vi "set wave form.vi"(10 "channels (0)":string[](array[string])=["0"], 11 "device (1)":i16=1) -> (0 "plot labels":T3, 1 "last value":dbl[](array[numeric]) format="%.2f", 2 "waveforms":T4 format="%.2f", 3 "SD method out":T2={"method array"=[], "Method Description"="", "data frequency"=1200, "repeat period"=2400} {"method array"."offset" format="%.2f"; "method array"."amplitude" format="%.2f"; "method array"."cycles/repeat period" min=1})   [LabVIEW 2010]
uses:
  wavecluster.ctl
  SDMethod.ctl
  plot labels.ctl
panel:
  in  "zoom control":T1(ring)=enum."Show repeat period"
  out "Time between Cursors":dbl format="%.4f"
  in  "show cycles":u32=1 min=1
  out "actual ticks per second":sgl format="%.8f"
  out "tick length":sgl=0.8333334 format="%.8f"
  in  "SD method default":T2 {"method array"."offset" format="%.2f"; "method array"."amplitude" format="%.2f"; "method array"."cycles/repeat period" min=1}
  out "channel label":string
  out "ticks/cycle":sgl=inf format="%.2f"
  out "integer":bool
  out "channel frequency":sgl format="%.8f"
  out "overall frequency":sgl=0.5 format="%.8f"
  in  "color":u32[](array[colorbox])=[255, 16711680, 52275, 16776960, 16750848, 16724991, 65535, 16777215]
  in  "load method":bool
  in  "save method":bool
  in  "SD method":T2={"method array"=[], "Method Description"="", "data frequency"=1200, "repeat period"=2400} {"method array"."waveform" items=["none", "one", "two", "3", "4", "5", "6", "7"]; "method array"."offset" format="%.2f"; "method array"."amplitude" format="%.2f"; "method array"."cycles/repeat period" min=1}
  in  "stop":bool
  out "graph":cluster{i32, sgl, "waveforms out":sgl[][]}(graph)={0, 0.00083333335, "waveforms out"=[]}
  # "ms"
  # "hz"
  # "ticks"
  # "hz"
  # "ms"
  # "hz"
  # "ticks"
  # "hz"
  # "ticks"
  # "ticks"
  # "volts"
  # "volts"
  # "ticks"
  # "hz"
  # "ticks"
  # "ticks"
  # "volts"
  # "volts"
  # "ticks"
  # "hz"
  # "ticks"
  # "ticks"
  # "volts"
  # "volts"
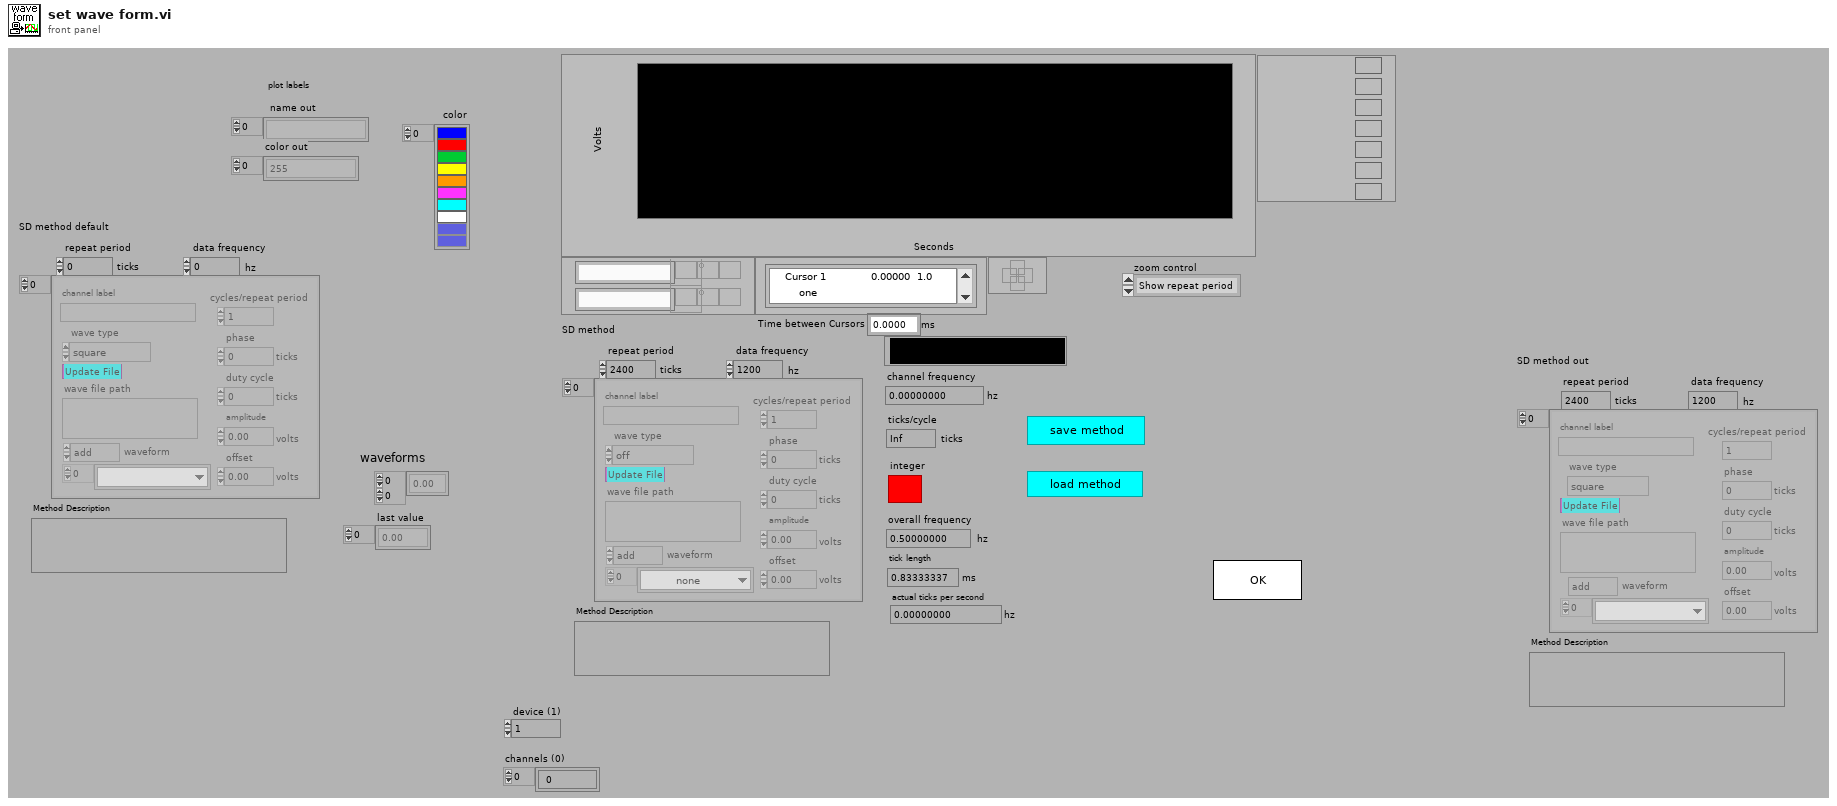
[diagram p1: front panel]
types:
  T1 = enum16{"Use zoom controls", "Show repeat period", "Show cycle"}
  T2 = typedef "SDMethod.ctl" = cluster{"method array":cluster{"wave type":enum16{"off", "square", "sine", "triangle", "sawtooth", "from file", "wavemaker", "flume pump"}, "cycles/repeat period":u32, "phase":i32, "duty cycle":u32, "wave file path":path, "amplitude":dbl, "channel label":string, "Update":bool, "offset":dbl, " waveform":u16[], "Function":enum16{"add", "multiply"}}[], "Method Description":string, "data frequency":u32, "repeat period":u32}
  T3 = typedef "plot labels.ctl" = cluster{"name out":string[], "color out":u32[]}
  T4 = typedef "wavecluster.ctl" = sgl[][]
  T5 = cluster{"wave type":enum16{"off", "square", "sine", "triangle", "sawtooth", "from file", "wavemaker", "flume pump"}, "cycles/repeat period":u32, "phase":i32, "duty cycle":u32, "wave file path":path, "amplitude":dbl, "channel label":string, "Update":bool, "offset":dbl, " waveform":u16[], "Function":enum16{"add", "multiply"}}[]
  T6 = cluster{"ticks per second used":sgl, "seconds per tick used":sgl, "timebase signal used":sgl, "timebase divisor used":i32}
  T7 = cluster{"wave type":enum16{"off", "square", "sine", "triangle", "sawtooth", "from file", "wavemaker", "flume pump"}, "cycles/repeat period":u32, "phase":i32, "duty cycle":u32, "wave file path":path, "amplitude":dbl, "channel label":string, "Update":bool, "offset":dbl, " waveform":u16[], "Function":enum16{"add", "multiply"}}
  T8 = enum16{"off", "square", "sine", "triangle", "sawtooth", "from file", "wavemaker", "flume pump"}
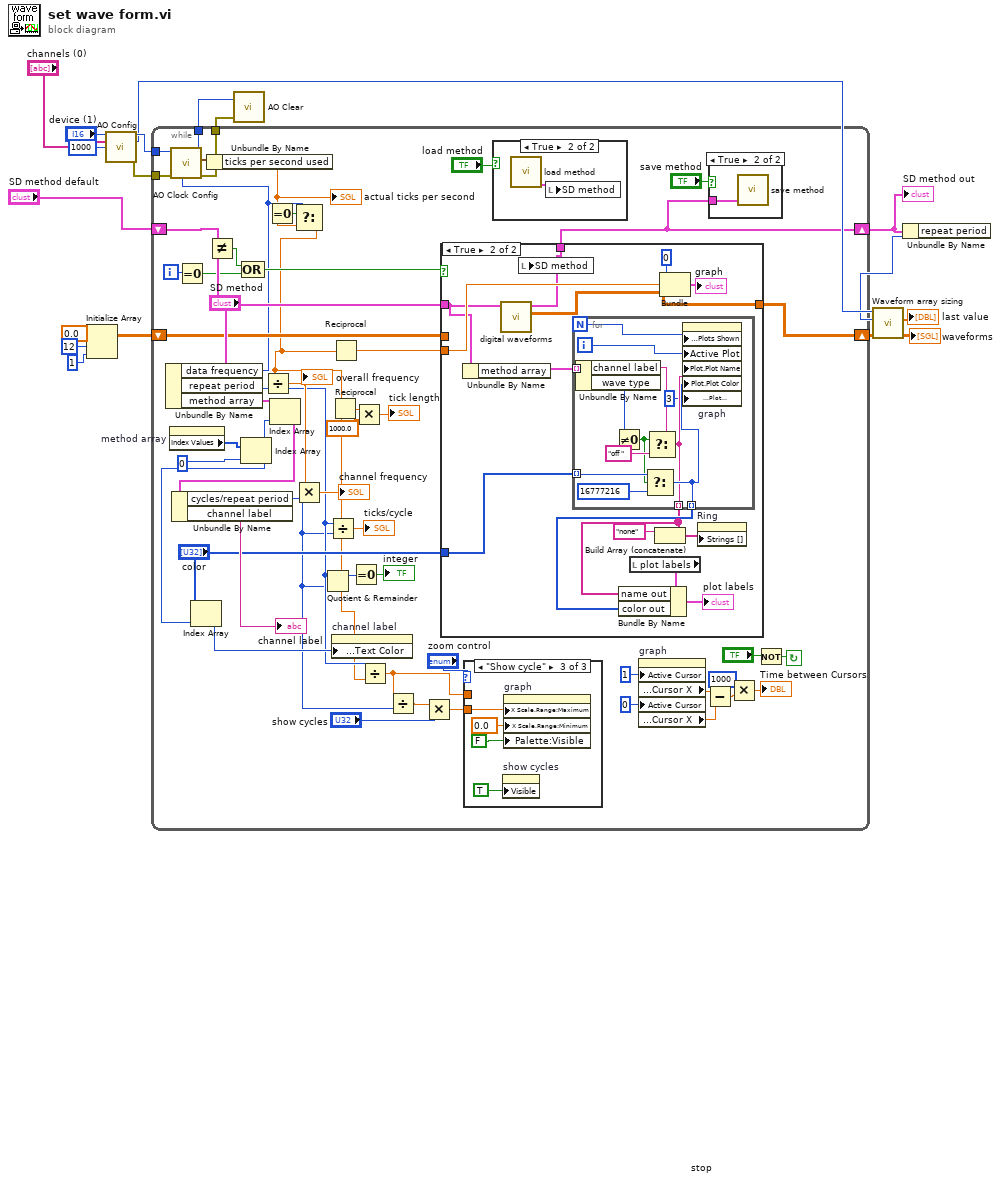
[diagram p0: block diagram]
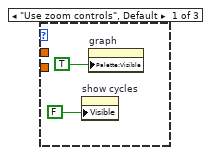
[diagram p2: hidden frame]
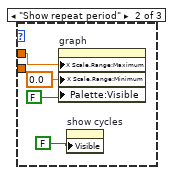
[diagram p3: hidden frame]
diagram:
  n1 = Initialize Array(sgl 0.0, 12, 1) -> (w16:sgl[][])
  n2 = call "AO Config.vi"("device (1)"="device (1)", "channels (0)"="channels (0)", "buffer size (1000 updates)"=1000) -> ("taskID"=w9:u32, "number of channels"=w3:u32, "error out"=w10:errorcluster)  [unwired: 10 in]
  n3 = while {
    tunnel: [w40] -> w7
    tunnel: [w41] -> w8
    tunnel: w9 -> [w44]
    tunnel: w10 -> [w42]
    shift-left: w16 -> [w58]
    shift-right: [w69] -> w4
    shift-left: "SD method default" -> [w64]
    shift-right: [w60] -> w14
    i -> [w68]
    stop <- w70 continue-if-true
    n4 = Unbundle By Name("SD method") -> ("data frequency"=w34:u32, "repeat period"=w39:u32, "method array"=w56:T5)
    n5 = property on="method array" class="Arr"() -> ("Index Values"=w29:u32[])  [unwired: 2 in, 2 out]
    n6 = call "AO Clock Config.vi"("ticks per second (-1: no change)"=w34, "error in (no error)"=w42, "task ID"=w44) -> ("error out"=w40:errorcluster, "actual rates used"=w43:T6, "task ID out"=w41:u32)  [unwired: 6 in]
    n7 = Equal To 0?(x=w68) -> (x = 0?=w59:bool)
    n8 = Unbundle By Name(w43) -> ("ticks per second used"=w33:sgl)
    "actual ticks per second" <- w33
    n9 = Not Equal?(x=w64, y="SD method") -> (x != y?=w67:bool)
    n10 = Index Array(array=w29, index=0) -> (element=w30:u32)
    n11 = Index Array(array="color", index=w30) -> (element=w49:u32)
    n12 = Compound Arithmetic op=OR(w67, w59) -> (w62:bool)
    n13 = Equal To 0?(x=w33) -> (x = 0?=w31:bool)
    n14 = Index Array(array=w56, index=w30) -> (element=w55:T7)
    n15 = Unbundle By Name(w55) -> ("cycles/repeat period"=w36:u32, "channel label"=→"channel label":string)
    n16 = Select(t=w34, s=w31, f=w33) -> (s? t:f=w32:sgl)
    n17 = Divide(x=w32, y=w39) -> (x/y=w45:sgl)
    "overall frequency" <- w45
    n18 = Multiply(x=w45, y=w36) -> (x*y=→"channel frequency":sgl)
    n19 = Quotient & Remainder(x=w39, y=w36) -> (x-y*floor(x/y)=w53:u32)  [unwired: 1 out]
    n20 = Divide(x=w39, y=w36) -> (x/y=→"ticks/cycle":dbl)
    n21 = Reciprocal(x=w32) -> (1/x=w47:sgl)
    n22 = Reciprocal(x=w32) -> (1/x=w63:sgl)
    n23 = property on="channel label" class="Str"("Text.Text Colors:Text Color"=w49) -> ()  [unwired: 2 in, 2 out]
    n24 = Equal To 0?(x=w53) -> (x = 0?=→"integer":bool)
    n25 = Multiply(x=w47, y=1000.0) -> (x*y=→"tick length":dbl)
    n26 = Divide(x=w39, y=w32) -> (x/y=w19:sgl)
    n27 = Divide(x=w19, y=w36) -> (x/y=w38:sgl)
    n28 = Multiply(x=w38, y="show cycles") -> (x*y=w20:sgl)
    n29 = case shown="True" w62 {
      tunnel: "SD method" -> [w84 w95]
      tunnel: [w85 w94] -> w69
      tunnel: w63 -> [_ w98]
      tunnel: w58 -> [w85 _]
      tunnel: [w84 w93] -> w60
      tunnel: "color" -> [_ w89]
      frame False {
      }
      frame True {
        n30 = Unbundle By Name(w95) -> ("method array"=w96:T5)
        n31 = call "digital waveforms.vi"("SD method in"=w95) -> ("waveforms out"=w94:T4, "SD method out"=w93:T2)  [unwired: 9 in]
        n32 = local write "SD method"(w93) -> ()
        n33 = for {
          N -> [w101]
          tunnel: w96 -> [w111] mode=indexing
          tunnel: w89 -> [w107] mode=indexing
          tunnel: [w105] -> w90 mode=indexing
          tunnel: [w104] -> w88 mode=indexing
          i -> [w102]
          n34 = Unbundle By Name(w111) -> ("channel label"=w109:string, "wave type"=w110:T8)
          n35 = Not Equal To 0?(x=w110) -> (x != 0?=w103:bool)
          n36 = Select(t=w107, s=w103, f=u32 16777216) -> (s? t:f=w105:u32)
          n37 = Select(t=w109, s=w103, f="off ") -> (s? t:f=w104:string)
          n38 = property on="graph" class="WFGraph (strict)"("Legend:Plots Shown"=w101, "Active Plot"=w102, "Plot.Plot Name"=w104, "Plot.Plot Color"=w105, "Plot.Plot Interpolation"=u8 3) -> ()  [unwired: 2 in, 2 out]
        }
        n39 = local read "plot labels"() -> (w92:T3)
        n40 = Bundle By Name(cluster=w92, "name out"=w88, "color out"=w90) -> (→"plot labels":T3)
        n41 = Build Array (concatenate)("none" ("Input Element"), w88) -> (w86:string[])
        n42 = Bundle(0, w98, "waveforms out"=w94) -> (→"graph":cluster{i32, sgl, "waveforms out":T4})  [unwired: 1 in]
        n43 = property on="Ring" class="Ring (strict)"("Strings []"=w86) -> ()  [unwired: 2 in, 2 out]
      }
    }
    n44 = case shown="\"Show cycle\"" "zoom control" {
      tunnel: w20 -> [_ _ w81]
      tunnel: w19 -> [_ w77 _]
      frame "Use zoom controls", Default {
        n45 = property on="show cycles" class="DigNum (strict)"("Visible"=FALSE) -> ()  [unwired: 2 in, 2 out]
        n46 = property on="graph" class="WFGraph (strict)"("Palette:Visible"=TRUE) -> ()  [unwired: 2 in, 2 out]
      }
      frame "Show repeat period" {
        n47 = property on="graph" class="WFGraph (strict)"("X Scale.Range:Maximum"=w77, "X Scale.Range:Minimum"=0.0, "Palette:Visible"=FALSE) -> ()  [unwired: 2 in, 2 out]
        n48 = property on="show cycles" class="DigNum (strict)"("Visible"=FALSE) -> ()  [unwired: 2 in, 2 out]
      }
      frame "Show cycle" {
        n49 = property on="show cycles" class="DigNum (strict)"("Visible"=TRUE) -> ()  [unwired: 2 in, 2 out]
        n50 = property on="graph" class="WFGraph (strict)"("X Scale.Range:Maximum"=w81, "X Scale.Range:Minimum"=0.0, "Palette:Visible"=FALSE) -> ()  [unwired: 2 in, 2 out]
      }
    }
    n51 = case shown="True" "load method" {
      frame False {
      }
      frame True {
        n52 = call "load method.vi"() -> ("SD method"=w82:T2)  [unwired: 10 in]
        n53 = local write "SD method"(w82) -> ()
      }
    }
    n54 = property on="graph" class="WFGraph (strict)"("Active Cursor"=u32 1, "Active Cursor"=u32 0) -> ("Cursor.Cursor Position:Cursor X"=w28:dbl, "Cursor.Cursor Position:Cursor X"=w27:dbl)  [unwired: 2 in, 2 out]
    n55 = Subtract(x=w28, y=w27) -> (x-y=w26:dbl)
    n56 = case shown="True" "save method" {
      tunnel: w60 -> [_ w83]
      frame False {
      }
      frame True {
        n57 = call "save method.vi"("SD method"=w83) -> ()  [unwired: 10 in]
      }
    }
    n58 = Multiply(x=1000, y=w26) -> (x*y=→"Time between Cursors":dbl)
    n59 = Not(x="stop") -> (.not. x?=w70:bool)
  }
  "SD method out" <- w14
  n60 = call "AO Clear.vi"("error in (no error)"=w7, "taskID in"=w8) -> ()  [unwired: 4 in, 2 out]
  n61 = Unbundle By Name(w14) -> ("repeat period"=w1:u32)
  n62 = call "Waveform array sizing.vi"("waveforms in"=w4, "repeat period (ticks)"=w1, "number of channels"=w3) -> ("waveforms out"=→"waveforms":T4, "last value"=→"last value":dbl[])  [unwired: 7 in]
